vi "PH_ImageCoG_Plotter.evt call set Pos Exp Values.vi"(0 "i ref in":refnum<vi>, 1 "Instance":string, 3 "expected value  x [Pix]":i32, 4 "expected value y [Pix]":i32, 5 "error in (no error)":errorcluster) -> (14 "i ref out":refnum<vi>, 19 "error out":errorcluster)   [LabVIEW 2014, in "PH_ImageCoG_Plotter.lvlib"]
doc: "This VI calls the event case \"SetPosExpValues\" by a simple call."
uses:
  PH_ImageCoG_Plotter.lvlib
  CS_Core/CSSystem/CoreLib/CoreLib.int 2 byte array.vi
  CS_Core/CSSystem/CoreLib/CoreLib.lvlib
  CS_Core/BaseProcess/BaseProcess.lvlib
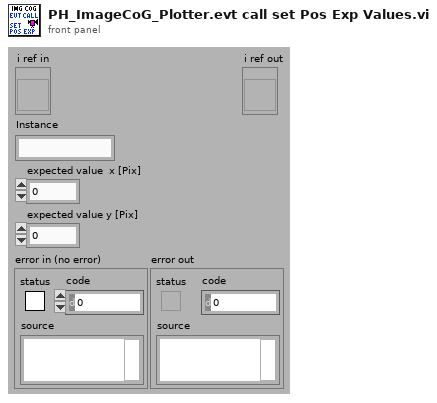
[diagram p1: front panel]
types:
  T1 = typedef "CoreDefs.rawDataType.ctl" = i8[]
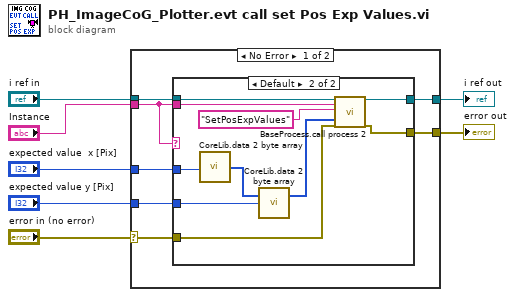
[diagram p0: block diagram]
diagram:
  n1 = case shown="No Error" "error in (no error)" {
    selector: "error in (no error)" -> [w11 w27]
    tunnel: [w14 w28] -> w6
    tunnel: [w13 w27] -> w5
    tunnel: "i ref in" -> [w12 w28]
    tunnel: "Instance" -> [w10 _]
    tunnel: "expected value y [Pix]" -> [w9 _]
    tunnel: "expected value  x [Pix]" -> [w8 _]
    frame No Error {
      n2 = case shown="Default" w10 {
        tunnel: [w16 w25] -> w14
        tunnel: [w15 w24] -> w13
        tunnel: w12 -> [w16 w23]
        tunnel: w10 -> [_ w22]
        tunnel: w11 -> [w15 w21]
        tunnel: w9 -> [_ w18]
        tunnel: w8 -> [_ w17]
        frame "N/A" {
        }
        frame Default {
          n3 = call-poly "CoreLib.data 2 byte array.vi"("i32"=w17) -> ("byteArray out"=w20:T1)  [unwired: 18 in]
          n4 = call-poly "CoreLib.data 2 byte array.vi"("byteArray"=w20, "i32"=w18) -> ("byteArray out"=w19:T1)  [unwired: 17 in]
          n5 = call "BaseProcess.call process 2.vi"("i ref in"=w23, "Object"=w22, "Selector"="SetPosExpValues", "Data"=w19, "error in (no error)"=w21) -> ("i ref out"=w25:refnum<vi>, "error out"=w24:errorcluster)  [unwired: 13 in]
        }
      }
    }
    frame Error {
    }
  }
  "i ref out" <- w6
  "error out" <- w5
